vi "Dashboard Main.vi"(0 "Controller Type":string(combo)) -> ()   [LabVIEW 2020]
uses:
  <vilib>/Utility/miscctls.llb/LVRowAndColumnTypeDef.ctl
  <vilib>/event_ctls.llb/eventvkey.ctl
  <vilib>/Rock Robotics/Network Tables/NT Read Numeric Array.vi
  <vilib>/Rock Robotics/WPI/Dashboard/WPI_DashboardLogging Global.vi
panel:
  in  "Camera Settings Right":T1={"Frame Rate"=30, "Compression"=30, "Size"=1, "DB Camera Config"=FALSE} {"Frame Rate" scale=1.0..30.0; "Compression" scale=100.0..-1.0; "Size" items=["640x480", "320x240", "160x120"]}
  in  "Camera Name Right":string(combo)="No Camera Selection"
  out "Camera Perf":string
  in  "Camera Settings":T1={"Frame Rate"=30, "Compression"=30, "Size"=1, "DB Camera Config"=FALSE} {"Frame Rate" scale=1.0..30.0; "Compression" scale=100.0..-1.0; "Size" items=["640x480", "320x240", "160x120"]}
  in  "TCP":refnum<k5>
  in  "Rec Mode":enum32{"Stop", "Record", "Playback"}(radio)
  out "Robot IP":string
  out "Image Message":string="Timeout in Camera Communications"
  in  "Dashboard Tab":T2(tab)
  in  "Select Auto":string(combo)="Select Autonomous ..."
  out "NT Connection":bool
  out "MotorChart R":cluster{"Numeric":dbl, "Numeric":dbl}(graph)
  out "MotorChart L":cluster{"Numeric":dbl, "Numeric":dbl}(graph)
  out "MotorSliders R":cluster{"MotorSlide1":dbl, "MotorSlide2":dbl} {"MotorSlide2" scale=-1.0..1.0 scale format="%#_2e"; "MotorSlide1" scale=-1.0..1.0 scale format="%#_2e"}
  out "MotorSliders L":cluster{"MotorSlide1":dbl, "MotorSlide2":dbl} {"MotorSlide2" scale=-1.0..1.0 scale format="%#_2e"; "MotorSlide1" scale=-1.0..1.0 scale format="%#_2e"}
  out "Gyro":dbl(knob) scale=0.0..360.0
  out "JS1 Z":dbl(slide) scale=-1.0..1.0 scale format="%#_2e"
  out "JS1 Graph":cluster{"X":dbl, "Y":dbl}[](graph)
  out "JS1 Buttons":T3
  out "JS2 Z":dbl(slide) scale=-1.0..1.0 scale format="%#_2e"
  out "JS2 Graph":cluster{"X":dbl, "Y":dbl}[](graph)
  out "JS2 Buttons":T3
  out "Mode":T4(ring)=enum."Auto Disabled"
  out "Right Camera Perf":cluster{"Bandwidth (Mbps)":dbl, "FPS":dbl}
  out "Camera Image Right":T5(plugin-control)
  in  "DB/String 9":string
  in  "DB/String 8":string
  in  "DB/String 7":string
  in  "DB/String 6":string
  in  "DB/String 5":string
  in  "DB/String 4":string
  in  "DB/String 3":string
  in  "DB/String 2":string
  in  "DB/String 1":string
  in  "DB/String 0":string
  in  "DB/Slider 0":dbl(slide) scale=0.0..5.0
  in  "DB/Slider 1":dbl(slide) scale=0.0..5.0
  in  "DB/Slider 2":dbl(slide) scale=0.0..5.0
  in  "DB/Slider 3":dbl(slide) scale=0.0..5.0
  out "DB/LED 3":bool
  out "DB/LED 2":bool
  out "DB/LED 1":bool
  out "DB/LED 0":bool
  in  "DB/Button 3":bool
  in  "DB/Button 2":bool
  in  "DB/Button 1":bool
  in  "DB/Button 0":bool caption="New Name"
  out "Controller Verification":string
  in  "Test Slider":dbl(slide) scale=0.0..100.0 scale format="%#_3g"
  in  "On/Off":bool caption="Solenoid"
  in  "Test Name":u16(ring) items=["Select the test to run..."]
  in  "Test Tree":string(tree)
  in  "Motor":cluster{"Value":dbl, "Enable":bool} {"Value" scale=-1.0..1.0 scale format="%#_3g"}
  out "Progress":T6 {"Test Progress" scale=0.0..100.0}
  in  "Rev/Fwd":cluster{"Forward":bool, "Reverse":bool}
  in  "Test Ring":u16(ring) items=["Monochrome", "Color"]
  out "Cmd Status":string
  in  "Execute Command":bool
  in  "Command Params":string[][](table)
  in  "Command Selection":i32(listbox)
  in  "CheckList":i32(listbox)
  out "Tree":string(tree)
  out "Camera Image":T5(plugin-control)
  out "Background":bool
  in  "Camera Name":string(combo)="No Camera Selection"
  # "HW"
  # "HW"
  # "Joysticks"
  # "Drive Motors"
  # "Front"
  # "Right"
  # "Left"
  # "Back"
  # "This tab is a great place for autonomous settings and robot-specific values.\nPlace controls and indicators inside this tab and match name to\nDashboard Variables on robot. You can also delete this comment."
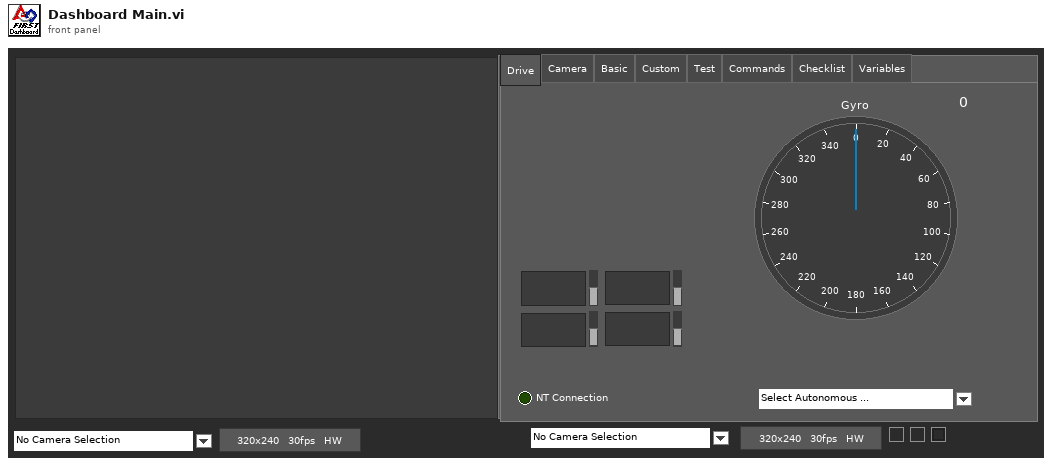
[diagram p1: front panel]
types:
  T1 = cluster{"Frame Rate":i32, "Compression":i32, "Size":u16, "DB Camera Config":bool}
  T2 = enum32{"Drive", "Camera", "Basic", "Custom", "Test", "Commands", "Checklist", "Variables"}
  T3 = cluster{bool, bool, bool, bool, bool, bool, bool, bool, bool, bool, bool, bool}
  T4 = enum8{"Tele-Op Disabled", "Tele-Op Enabled", "Auto Disabled", "Auto Enabled", "Test Disabled", "Test Enabled", "Disconnected", "No Code", "E-Stop"}
  T5 = typedef "IMAQ Image.ctl" = refnum<image>
  T6 = cluster{"Test Progress":u8, "Test Progress Text":string}
  T7 = cluster{"Save Path":path, "Interval (s)":dbl, "Keep":i32}
  T8 = typedef "Image Type" = u32
  T9 = cluster{"IDs":cluster{"RPC field ID":u16, "Unique ID":u16}, "String":string}
  T10 = cluster{"Error Strings":string, "Disable Counts":cluster{u16, u16}, "Rail Faults":cluster{u16, u16, u16}, "Robot IP":string, "DB Mode":u8, "Event Info":cluster{"Name":string, "Type":u8, "Number":u16, "Replay":u8}}
  T11 = cluster{"Storage":cluster{"Disk Free":u64, "RAM Block":u32, "RAM free":u32}, "CPU Utilization":cluster{"CPU % ISR":sgl, "CPU % Time Crit":sgl, "CPU % Timed Str":sgl, "CPU % High":sgl, "CPU % Above":sgl, "CPU % Normal":sgl, "CPU % Low":sgl}, "CAN":cluster{"% Bus Utilization":sgl, "Bus Off Cnt":u32, "TX_FIFO Full Cnt":u32, "Receive Error Cnt":u8, "Transmit Error Cnt":u8}, "HID":cluster{"HID Outputs":u32, "Rumble Low":u16, "Rumble High":u16}[]}
  T12 = cluster{"Status bits":cluster{"Test Mode":bool, "Autonomous":bool, "Enabled":bool, "Code Start":bool, "Brownout":bool, "Reserved 2":bool, "Reserved 3":bool, "E-Stop":bool}, "Code Trace":cluster{"Disabled":bool, "TeleOp":bool, "Auto":bool, "Test":bool}, "Controller Type":enum16{"unknown", "cRIO", "roboRio"}, "Code?":enum16{"unknown", "noCode", "code"}, "Battery V":dbl}
  T13 = cluster{"Control Bits":cluster{"TestMode":bool, "Autonomous":bool, "Enabled":bool, "FMS Present":bool, bool, bool, bool, "E-Stop":bool}, "Team Station ":u8, "Countdown":sgl, "Joystick Values":cluster{"Axes":dbl[], "Buttons":bool[], "POVs":i16[]}[]}
  T14 = cluster{"Axes":dbl[], "Buttons":bool[], "POVs":i16[]}[]
  T15 = cluster{"Axes":dbl[], "Buttons":bool[], "POVs":i16[]}
  T16 = cluster{"Buttons[0]":bool, "Buttons[1]":bool, "Buttons[2]":bool, "Buttons[3]":bool, "Buttons[4]":bool, "Buttons[5]":bool, "Buttons[6]":bool, "Buttons[7]":bool, "Buttons[8]":bool, "Buttons[9]":bool, "Buttons[10]":bool, "Buttons[11]":bool}
  T17 = cluster{"Camera Image":refnum<vi>, "Dashboard Tab":refnum<vi>, "Background":refnum<vi>, "Rec Mode":refnum<vi>, "Test Slider":refnum<vi>, "On/Off ":refnum<vi>, "Test Ring":refnum<vi>, "Rev/Fwd":refnum<vi>, "Test Name":refnum<vi>, "Motor":refnum<vi>, "Progress":refnum<vi>, "CheckList":refnum<vi>, "Tree":refnum<vi>, "Test Tree":refnum<vi>, "Command Params":refnum<vi>, "Command Selection":refnum<vi>, "Execute Command":refnum<vi>, "Cmd Status":refnum<vi>, "Camera Settings":refnum<vi>, "Camera Name":refnum<vi>, "Camera Perf":refnum<vi>, "Camera Settings Right":refnum<vi>, "Camera Name Right":refnum<vi>, "Camera Image Right":refnum<vi>}
  T18 = cluster{"Global Rectangle":i32[], "Contours":cluster{"Contour Type":u32, "ROI Type":u32, "Points":i32[]}[]}
  T19 = cluster{"Camera Name":string, string, "Saved DB Images Info":cluster{"Save Path":path, "Interval (s)":dbl, "Keep":i32}}
  T20 = cluster{"Camera Name Right":string, string, "Saved DB Images Info":cluster{"Save Path":path, "Interval (s)":dbl, "Keep":i32}}
  T21 = cluster{"Operation":enum16{"Update", "Clear"}, "Color Box":u32}[]
  T22 = typedef "eventvkey.ctl" = enum16{"ASCII", "Enter", "Return", "Shift", "Ctrl", "Alt", "Cmd", "Opt", "Caps", "NumLock", "Clear", "Break", "Up", "Down", "Left", "Right", "Insert", "Delete", "Home", "End", "PageUp", "PageDown", "Escape", "Help", "Pause", "ScrollLock", "F1", "F2", "F3", "F4", "F5", "F6", "F7", "F8", "F9", "F10", "F11", "F12", "F13", "F14", "F15", "F16", "F17", "F18", "F19", "F20", "F21", "F22", "F23", "F24", "Play", "VolumeUp", "VolumeDown", "Mute", "Two Byte Char"}
  T23 = cluster{"Image Size":bool, "Image Type":bool, "Pixel Value":bool, "ROI Information":bool, "Zoom Factor":bool}
  T24 = cluster{"Operation":enum16{"Update", "Clear"}, "Color Box":u32}
  T25 = typedef "LVRowAndColumnTypeDef.ctl" = cluster{"Row":i32, "Column":i32}
  T26 = cluster{"Shift":bool, "Ctrl":bool, "Alt":bool, "Cmd":bool, "Opt":bool}
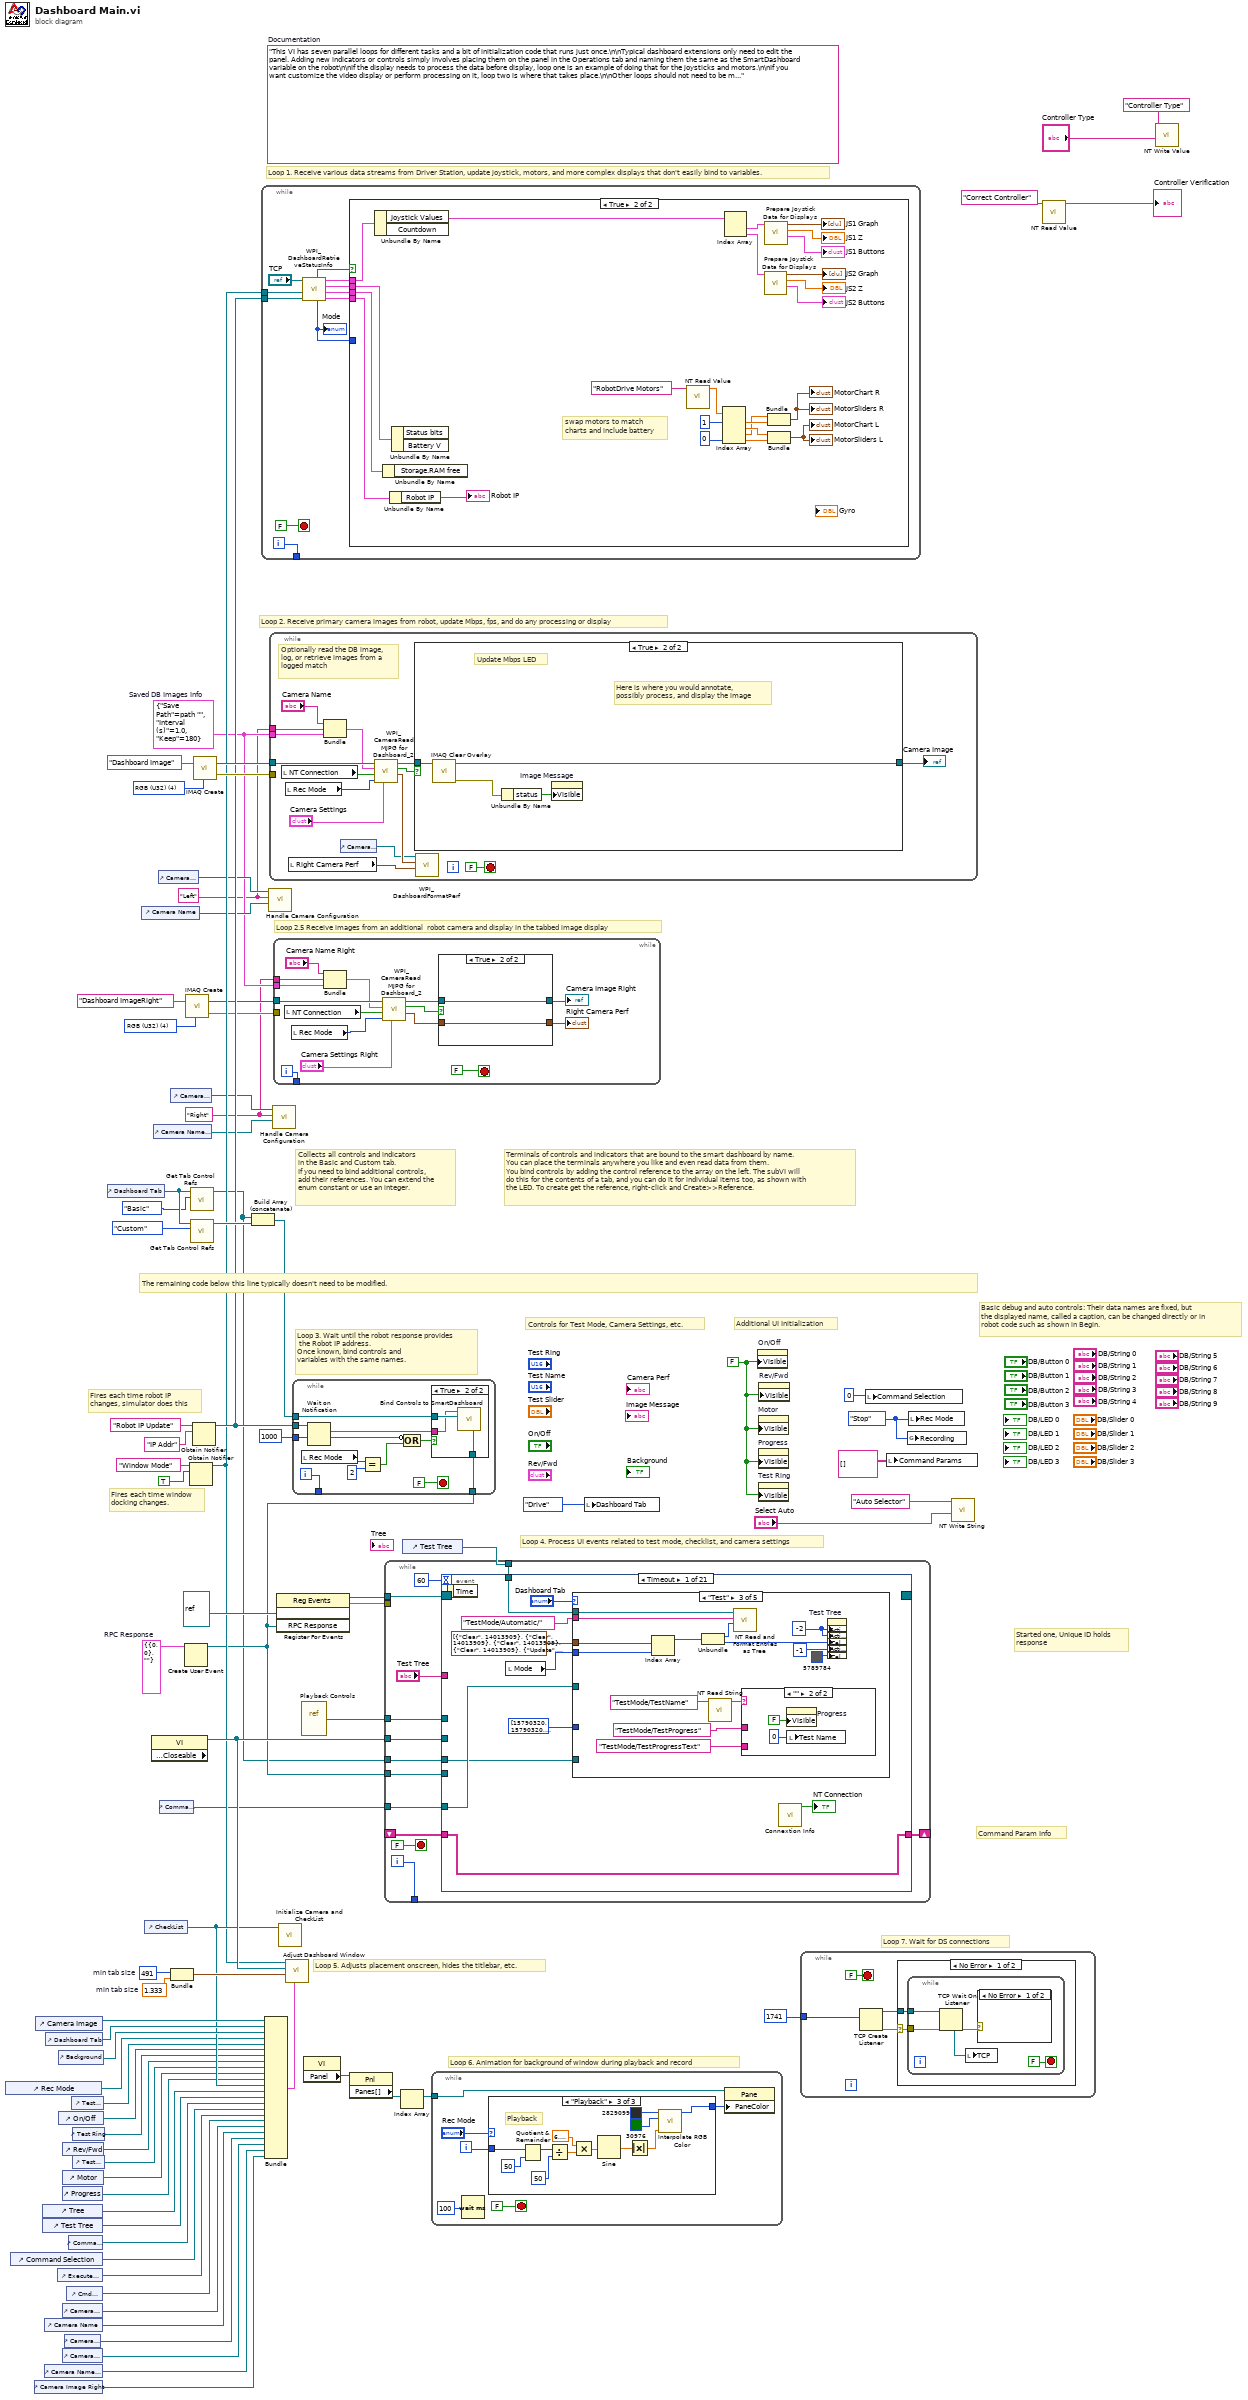
[diagram p0: block diagram]
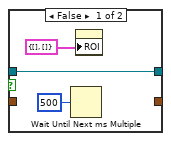
[diagram p2: hidden frame]
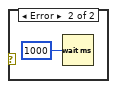
[diagram p3: hidden frame]
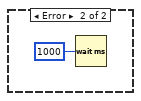
[diagram p4: hidden frame]
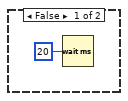
[diagram p5: hidden frame]
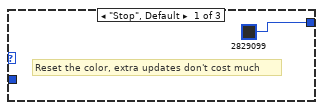
[diagram p6: hidden frame]
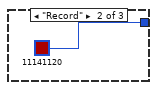
[diagram p7: hidden frame]
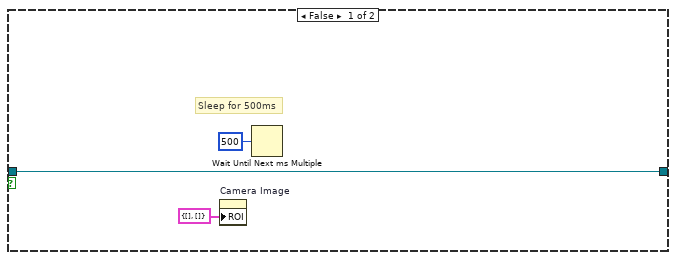
[diagram p9: hidden frame]
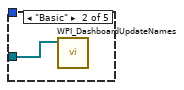
[diagram p11: hidden frame]
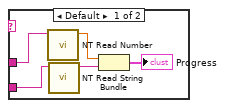
[diagram p12: hidden frame]
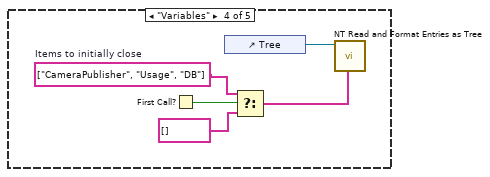
[diagram p13: hidden frame]
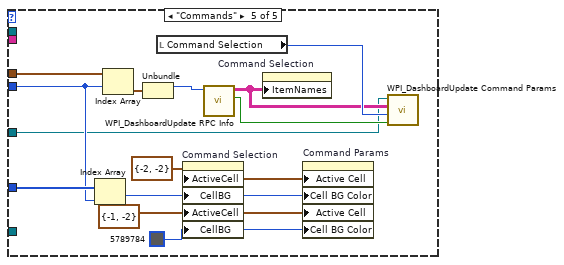
[diagram p14: hidden frame]
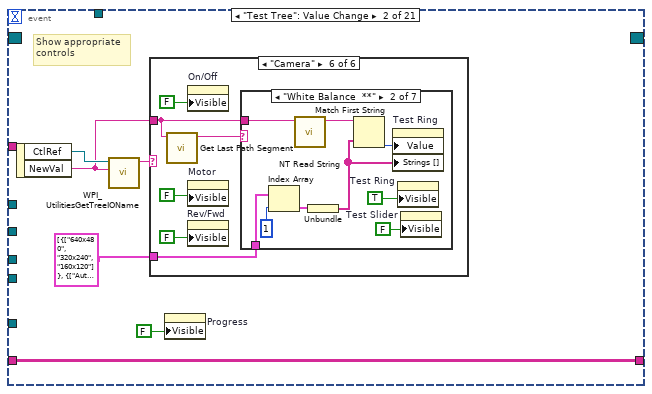
[diagram p15: hidden frame]
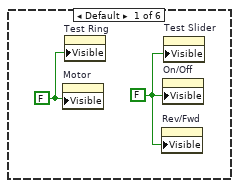
[diagram p16: hidden frame]
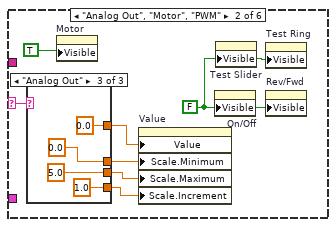
[diagram p17: hidden frame]
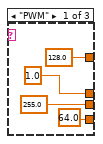
[diagram p18: hidden frame]
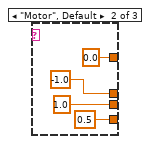
[diagram p19: hidden frame]
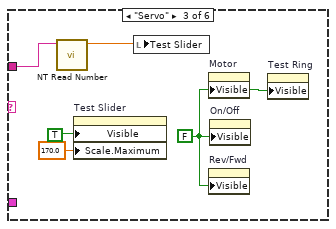
[diagram p20: hidden frame]
diagram:
  w7 = T7 {"Save Path"=path "", "Interval (s)"=1.0, "Keep"=180}  # Saved DB Images Info
  w6 = "Right"
  w5 = "Left"
  w17 = T8 4 items=["Grayscale (U8)", "Grayscale (I16)", "Grayscale (SGL)", "Complex (CSG)", "RGB (U32)", "HSL (U32)", "RGB (U64)"] ("Image Type")
  w33 = T9 {"IDs"={"RPC field ID"=0, "Unique ID"=0}, "String"=""}  # RPC Response
  w56 = 491  # min tab size
  w55 = 1.333  # min tab size
  w63 = enum32{"Stop", "Record", "Playback"}."Stop" ("Rec Mode")
  w40 = FALSE ("Visible")
  (unwired) "This VI has seven parallel loops for different tasks and a bit of initialization code that runs just once.\n\nTypical dashboard extensions only need to edit the panel. Adding new indicators or controls simply involves placing them on the panel in the Operations tab and naming them the same as the SmartDashboard variable on the robot\n\nIf the display needs to process the data before display, loop one is an example of doing that for the joysticks and motors.\n\nIf you want customize the video display or perform processing on it, loop two is where that takes place.\n\nOther loops should not need to be modified. They are pretty standard, and document the task they perform."  # Documentation
  w80 = T8 4 items=["Grayscale (U8)", "Grayscale (I16)", "Grayscale (SGL)", "Complex (CSG)", "RGB (U32)", "HSL (U32)", "RGB (U64)"] ("Image Type")
  # "Loop 2.5 Receive images from an additional  robot camera and display in the tabbed image display"
  # "Command Param Info"
  # "Started one, Unique ID holds\nresponse"
  # "Loop 7. Wait for DS connections"
  # "Basic debug and auto controls: Their data names are fixed, but\nthe displayed name, called a caption, can be changed directly or in\nrobot code such as shown in Begin."
  # "Controls for Test Mode, Camera Settings, etc."
  # "Additional UI Initialization"
  # "Loop 6. Animation for background of window during playback and record"
  # "Fires each time robot IP\nchanges, simulator does this"
  # "Fires each time window\ndocking changes."
  # "Collects all controls and indicators\nin the Basic and Custom tab.\nIf you need to bind additional controls,\nadd their references. You can extend the\nenum constant or use an integer."
  # "The remaining code below this line typically doesn't need to be modified."
  # "Loop 4. Process UI events related to test mode, checklist, and camera settings"
  # "Terminals of controls and indicators that are bound to the smart dashboard by name.\nYou can place the terminals anywhere you like and even read data from them.\nYou bind controls by adding the control reference to the array on the left. The subVI will\ndo this for the contents of a tab, and you can do it for individual items too, as shown with\nthe LED. To create get the reference, right-click and Create>>Reference."
  # "Loop 3. Wait until the robot response provides\n the Robot IP address.\nOnce known, bind controls and\nvariables with the same names."
  # "Loop 5. Adjusts placement onscreen, hides the titlebar, etc."
  # "Loop 1. Receive various data streams from Driver Station, update joystick, motors, and more complex displays that don't easily bind to variables."
  # "Loop 2. Receive primary camera images from robot, update Mbps, fps, and do any processing or display"
  n1 = control-ref of="Rec Mode"() -> (w46:refnum<vi>)
  n2 = control-ref of="Command Selection"() -> (w32:refnum<vi>)
  n3 = control-ref of="Camera Image Right"() -> (w10:refnum<vi>)
  n4 = control-ref of="Camera Image"() -> (w58:refnum<vi>)
  n5 = control-ref of="Tree"() -> (w50:refnum<vi>)
  n6 = control-ref of="Test Tree"() -> (w49:refnum<vi>)
  n7 = control-ref of="Camera Name"() -> (w23:refnum<vi>)
  n8 = control-ref of="Camera Name Right"() -> (w11:refnum<vi>)
  n9 = control-ref of="Dashboard Tab"() -> (w57:refnum<vi>)
  n10 = control-ref of="Execute Command"() -> (w34:refnum<vi>)
  n11 = control-ref of="Background"() -> (w53:refnum<vi>)
  n12 = control-ref of="On/Off"() -> (w44:refnum<vi>)
  n13 = control-ref of="Progress"() -> (w41:refnum<vi>)
  n14 = control-ref of="Camera Settings"() -> (w24:refnum<vi>)
  n15 = control-ref of="Camera Settings Right"() -> (w12:refnum<vi>)
  n16 = control-ref of="Rev/Fwd"() -> (w42:refnum<vi>)
  n17 = control-ref of="Motor"() -> (w47:refnum<vi>)
  n18 = control-ref of="Camera Perf"() -> (w22:refnum<vi>)
  n19 = control-ref of="Cmd Status"() -> (w28:refnum<vi>)
  n20 = control-ref of="Command Params"() -> (w35:refnum<vi>)
  n21 = control-ref of="Test Slider"() -> (w45:refnum<vi>)
  n22 = control-ref of="Test Ring"() -> (w43:refnum<vi>)
  n23 = control-ref of="Test Name"() -> (w48:refnum<vi>)
  n24 = control-ref of="Dashboard Tab"() -> (w61:refnum<vi>)
  n25 = control-ref of="Camera Name"() -> (w25:refnum<vi>)
  n26 = control-ref of="CheckList"() -> (w51:refnum<vi>)
  n27 = property class="VI" props=["Front Panel.Closeable"]() -> (reference out=w62:refnum<vi>)  [unwired: 2 in, 2 out]
  n28 = control-ref of="Camera Name Right"() -> (w13:refnum<vi>)
  n29 = control-ref of="Camera Settings"() -> (w26:refnum<vi>)
  n30 = control-ref of="Command Params"() -> (w27:refnum<vi>)
  n31 = control-ref of="Camera Settings Right"() -> (w14:refnum<vi>)
  n32 = Bundle("min tab size"=w56, "min tab size"=w55) -> (w54:cluster{"min tab size":i32, "min tab size":dbl})  [unwired: 1 in]
  n33 = Create User Event(user event datatype=w33) -> (user event=w29:refnum<user-event>)  [unwired: 1 in, 1 out]
  n34 = call "IMAQ Create"("Image Name"="Dashboard ImageRight", "Image Type"=w17) -> ("New Image"=w16:T5, "error out"=w15:errorcluster)  [unwired: 2 in, 1 out]
  n35 = Obtain Notifier(name (unnamed)="Window Mode", notification data type=TRUE) -> (notifier out=w38:refnum<notifier>)  [unwired: 2 in, 2 out]
  n36 = call <vilib>:"Get Tab Control Refs.vi"("Page Index"=T2."Basic" ("Dashboard Tab"), "TabControl in"=w61) -> ("ControlsOnPage"=w21:refnum<vi>[])  [unwired: 9 in]
  n37 = call <vilib>:"Get Tab Control Refs.vi"("Page Index"=T2."Custom" ("Dashboard Tab"), "TabControl in"=w61) -> ("ControlsOnPage"=w60:refnum<vi>[])  [unwired: 9 in]
  n38 = Obtain Notifier(name (unnamed)="Robot IP Update", notification data type="IP Addr" ("name (unnamed)")) -> (notifier out=w39:refnum<notifier>)  [unwired: 2 in, 2 out]
  n39 = call "IMAQ Create"("Image Name"="Dashboard Image", "Image Type"=w80) -> ("New Image"=w78:T5, "error out"=w77:errorcluster)  [unwired: 2 in, 1 out]
  n40 = Build Array (concatenate)(w21, w60) -> (w59:refnum<vi>[])
  n41 = while {
    tunnel: [w90] -> _
    tunnel: w39 -> [w84]
    tunnel: w38 -> [w81]
    i -> [w90]
    stop <- FALSE stop-if-true
    n42 = call <vilib>:"WPI_DashboardRetrieveStatusInfo.vi"("Binding Refnum"=w84, "Window Mode Notifier"=w81, "TCP Cnx"="TCP") -> ("Power and Errors"=w85:T10, "Robot Metrics"=w88:T11, "Status Info"=w89:T12, "Control Info"=w86:T13, "Robot Mode"=w83:T4, "Process?"=w87:bool)  [unwired: 3 in]
    "Mode" <- w83
    n43 = case shown="True" w87 {
      tunnel: w89 -> [_ w116]
      tunnel: w88 -> [_ w115]
      tunnel: w86 -> [_ w114]
      tunnel: w85 -> [_ w113]
      tunnel: w83 -> [_ _]
      frame False {
        n44 = Wait (ms)(milliseconds to wait=u32 20) -> ()  [unwired: 1 out]
      }
      frame True {
        # "swap motors to match\ncharts and include battery"
        n45 = Unbundle By Name(w114) -> ("Joystick Values"=w104:T14)  [unwired: 1 out]
        n46 = Unbundle By Name(w115) -> ()  [unwired: 1 out]
        n47 = Unbundle By Name(w113) -> ("Robot IP"=→"Robot IP":string)
        n48 = Unbundle By Name(w116) -> ()  [unwired: 2 out]
        n49 = call-poly <vilib>:"NT Read Value.vi"("Name"="RobotDrive Motors") -> ("Numeric Array"=w94:dbl[])  [unwired: 9 in, 1 out]
        n50 = Index Array(array=w94, index #1=1, index #4=0) -> (element #1=w108:dbl, element #2=w109:dbl, element #3=w107:dbl, element #4=w112:dbl)  [unwired: 2 in]
        n51 = Index Array(array=w104) -> (element #1=w103:T15, element #2=w99:T15)  [unwired: 2 in]
        n52 = call "Prepare Joystick Data for Displays.vi"("Joystick Values"=w99) -> ("Buttons"=→"JS2 Buttons":T16, "Z Axis"=→"JS2 Z":dbl, "Cartesian Data"=→"JS2 Graph":cluster{"X axis":dbl, "X axis":dbl}[])  [unwired: 8 in]
        n53 = call "Prepare Joystick Data for Displays.vi"("Joystick Values"=w103) -> ("Buttons"=→"JS1 Buttons":T16, "Z Axis"=→"JS1 Z":dbl, "Cartesian Data"=→"JS1 Graph":cluster{"X axis":dbl, "X axis":dbl}[])  [unwired: 8 in]
        n54 = Bundle("Numeric"=w107, "Numeric"=w108) -> (→"MotorChart R" →"MotorSliders R":cluster{"Numeric":dbl, "Numeric":dbl})  [unwired: 1 in]
        n55 = Bundle("Numeric"=w109, "Numeric"=w112) -> (→"MotorChart L" →"MotorSliders L":cluster{"Numeric":dbl, "Numeric":dbl})  [unwired: 1 in]
      }
    }
  }
  n56 = Bundle("Camera Image"=w58, "Dashboard Tab"=w57, "Background"=w53, "Rec Mode"=w46, "Test Slider"=w45, "On/Off"=w44, "Test Ring"=w43, "Rev/Fwd"=w42, "Test Name"=w48, "Motor"=w47, "Progress"=w41, "CheckList"=w51, "Tree"=w50, "Test Tree"=w49, "Command Params"=w35, "Command Selection"=w32, "Execute Command"=w34, "Cmd Status"=w28, "Camera Settings"=w24, "Camera Name"=w23, "Camera Perf"=w22, "Camera Settings Right"=w12, "Camera Name Right"=w11, "Camera Image Right"=w10) -> (w52:T17)  [unwired: 1 in]
  n57 = call "Handle Camera Configuration.vi"("CameraNameRef"=w25, "Display Name"=w5, "ClusterRef"=w26) -> ()  [unwired: 9 in]
  n58 = while {
    tunnel: w78 -> [w130]
    tunnel: w77 -> [_]
    tunnel: w7 -> [w123]
    tunnel: w5 -> [w120]
    stop <- FALSE stop-if-true
    # "Optionally read the DB image,\nlog, or retrieve images from a\nlogged match"
    n59 = local read "NT Connection"() -> (w124:bool)
    n60 = local read "Rec Mode"() -> (w127:enum32{"Stop", "Record", "Playback"})
    n61 = local read "Right Camera Perf"() -> (w118:cluster{"Bandwidth (Mbps)":dbl, "FPS":dbl})
    n62 = Bundle("Camera Name"="Camera Name", w120, "Saved DB Images Info"=w123) -> (w122:T19)  [unwired: 1 in]
    n63 = control-ref of="Camera Perf"() -> (w117:refnum<vi>)
    n64 = call <vilib>:"WPI_CameraRead MJPG for Dashboard_2.vi"("Camera Settings"="Camera Settings", "Rec Mode"=w127, "NT Connection"=w124, "Capture Info"=w122, "Image in"=w130) -> ("perf info"=w119:cluster{"Bandwidth (Mbps)":dbl, "fps":dbl}, "Active"=w128:bool, "Image\\ out"=w129:T5)  [unwired: 4 in]
    n65 = case shown="True" w128 {
      tunnel: w129 -> [w133 w136]
      tunnel: [w133 w135] -> w125
      frame False {
        # "Sleep for 500ms"
        n66 = property on="Camera Image" class="ImageControl"("ROI"=T18 {"Global Rectangle"=[], "Contours"=[]}) -> ()  [unwired: 2 in, 2 out]
        n67 = Wait Until Next ms Multiple(millisecond multiple=u32 500) -> ()  [unwired: 1 out]
      }
      frame True {
        # "Here is where you would annotate,\npossibly process, and display the image"
        # "Update Mbps LED"
        n68 = call "IMAQ Clear Overlay"("Image"=w136) -> ("error out"=w137:errorcluster, "Image Out"=w135:T5)  [unwired: 2 in, 7 out]
        n69 = Unbundle By Name(w137) -> ("status"=w138:bool)
        n70 = property on="Image Message" class="Str"("Visible"=w138) -> ()  [unwired: 2 in, 2 out]
      }
    }
    "Camera Image" <- w125
    n71 = call <vilib>:"WPI_DashboardFormatPerf.vi"("Right Camera Perf"=w118, "Performance"=w119, "String in"=w117) -> ()  [unwired: 9 in]
  }
  n72 = call "Handle Camera Configuration.vi"("CameraNameRef"=w13, "Display Name"=w6, "ClusterRef"=w14) -> ()  [unwired: 9 in]
  n73 = while {
    tunnel: w16 -> [w153]
    tunnel: w15 -> [_]
    tunnel: [w148] -> _
    tunnel: w7 -> [w144]
    tunnel: w6 -> [w141]
    i -> [w148]
    stop <- FALSE stop-if-true
    n74 = local read "NT Connection"() -> (w145:bool)
    n75 = local read "Rec Mode"() -> (w152:enum32{"Stop", "Record", "Playback"})
    n76 = Bundle("Camera Name Right"="Camera Name Right", w141, "Saved DB Images Info"=w144) -> (w143:T20)  [unwired: 1 in]
    n77 = call <vilib>:"WPI_CameraRead MJPG for Dashboard_2.vi"("Camera Settings"="Camera Settings Right", "Rec Mode"=w152, "NT Connection"=w145, "Capture Info"=w143, "Image in"=w153) -> ("perf info"=w139:cluster{"Bandwidth (Mbps)":dbl, "fps":dbl}, "Active"=w147:bool, "Image\\ out"=w150:T5)  [unwired: 4 in]
    n78 = case shown="True" w147 {
      tunnel: w150 -> [w155 w158]
      tunnel: [w155 w158] -> w146
      tunnel: [_ w157] -> w140
      tunnel: w139 -> [_ w157]
      frame False {
        n79 = Wait Until Next ms Multiple(millisecond multiple=u32 500) -> ()  [unwired: 1 out]
        n80 = property on="Camera Image Right" class="ImageControl"("ROI"=T18 {"Global Rectangle"=[], "Contours"=[]}) -> ()  [unwired: 2 in, 2 out]
      }
      frame True {
      }
    }
    "Camera Image Right" <- w146
    "Right Camera Perf" <- w140
  }
  n81 = register-events(refnum<vi> refnum, w29) -> (reference out=w67:refnum<event-registration>, error out=w66:errorcluster)  [unwired: 2 in]
  n82 = call "Initialize Camera and CheckList.vi"("ListBox in"=w51) -> ()  [unwired: 11 in]
  n83 = call "Adjust Dashboard Window.vi"("Sizing Refnums"=w52, "Size Constraints"=w54, "VI"=w62, "WIn Mode"=w38) -> ()  [unwired: 8 in]
  n84 = while {
    tunnel: w59 -> [w170]
    tunnel: w39 -> [w168]
    tunnel: [w166] -> _
    tunnel: u32 1000 ("milliseconds to wait") -> [w165]
    tunnel: w29 -> [w159]
    i -> [w166]
    stop <- FALSE stop-if-true
    n85 = local read "Rec Mode"() -> (w161:enum32{"Stop", "Record", "Playback"})
    n86 = Wait on Notification(notifier=w168, timeout in ms (-1)=w165) -> (notification=w167:string, timed out?=w163:bool)  [unwired: 2 in, 2 out]
    n87 = Equal?(x=w161, y=u16 2 ("Rec Mode")) -> (x = y?=w162:bool)
    n88 = Compound Arithmetic op=OR(invert w163, w162) -> (w164:bool)
    n89 = case shown="True" w164 {
      tunnel: w170 -> [_ w173]
      tunnel: w167 -> [_ w172]
      tunnel: w159 -> [_ w171]
      frame False {
      }
      frame True {
        n90 = call <vilib>:"Bind Controls to SmartDashboard.vi"("RPC ref"=w171, "Bound Control Refs"=w173, "Server IP Address"=w172) -> ()  [unwired: 9 in]
      }
    }
  }
  n91 = vi-ref "Playback Controls.vi"() -> (w68:refnum<vi>)
  n92 = property class="VI"() -> ("Panel"=w70:refnum<vi>)  [unwired: 2 in, 2 out]
  n93 = property class="Pnl"(reference=w70) -> ("Panes[]"=w71:refnum<vi>[])  [unwired: 1 in, 2 out]
  n94 = Index Array(array=w71) -> (element=w69:refnum<vi>)  [unwired: 1 in]
  n95 = control-ref of="Test Tree"() -> (w72:refnum<vi>)
  n96 = while {
    tunnel: [w183] -> _
    tunnel: w72 -> [w182]
    tunnel: w68 -> [w181]
    tunnel: w67 -> [w180]
    tunnel: w66 -> [_]
    tunnel: w62 -> [w179]
    tunnel: w29 -> [w178]
    tunnel: w27 -> [w177]
    shift-right: [w176] -> _
    shift-left: _ -> [w175]
    tunnel: w21 -> [w174]
    i -> [w183]
    stop <- FALSE stop-if-true
    n97 = event shown="[0] Timeout" {
      selector: w180 -> [_ _ _ _ _ _ _ _ _ _ _ _ _ _ _ _ _ _ _ _ _]
      dyn-events: [_ _ _ _ _ _ _ _ _ _ _ _ _ _ _ _ w443 _ _ _ _] -> _
      timeout: u32 60 ("milliseconds to wait") -> [_ _ _ _ _ _ _ _ _ _ _ _ _ _ _ _ _ _ _ _ _]
      tunnel: w182 -> [w195 _ _ _ _ _ _ _ _ _ _ _ _ _ _ _ _ _ _ _ _]
      tunnel: "Test Tree" -> [_ _ _ _ _ _ _ _ _ _ _ w410 w418 w420 w424 w432 _ _ _ _ _]
      tunnel: w181 -> [_ _ _ _ _ _ _ _ _ _ _ _ _ _ _ _ w445 _ w463 _ _]
      tunnel: w179 -> [_ _ _ _ _ _ _ _ _ _ _ _ _ _ _ _ w441 _ _ _ _]
      tunnel: w178 -> [_ _ _ _ _ _ _ _ _ _ _ _ _ _ _ _ w439 _ _ _ _]
      tunnel: w177 -> [w190 _ _ _ _ _ w361 _ _ _ _ _ _ _ _ _ _ _ _ _ _]
      tunnel: [w189 w238 w340 w345 w354 w358 w359 w368 w378 w385 w397 w409 w416 w419 w423 w431 w438 w458 w460 w464 w477] -> w176
      tunnel: w175 -> [w189 w238 w340 w345 w354 w358 w359 _ _ w385 w397 w409 w416 w419 w423 w431 w438 w458 w460 w464 w477]
      tunnel: w174 -> [w187 _ _ _ _ _ _ _ _ _ _ _ _ _ _ _ _ _ _ _ _]
      event Timeout {
        n98 = event-data() -> ()  [unwired: 1 in, 1 out]
        n99 = local read "Mode"() -> (w192:T4)
        n100 = case shown="\"Test\"" "Dashboard Tab" {
          tunnel: w195 -> [_ _ w211 _ _]
          tunnel: "TestMode/Automatic/" ("Name Pattern") -> [_ _ w210 _ _]
          tunnel: T21 [{"Operation"=enum."Clear", "Color Box"=14013909}, {"Operation"=enum."Clear", "Color Box"=14013909}, {"Operation"=enum."Clear", "Color Box"=14013909}, {"Operation"=enum."Clear", "Color Box"=14013909}, {"Operation"=enum."Update", "Color Box"=14013909}, {"Operation"=enum."Update", "Color Box"=16777215}, {"Operation"=enum."Clear", "Color Box"=14013909}, {"Operation"=enum."Clear", "Color Box"=14013909}, {"Operation"=enum."Clear", "Color Box"=14013909}] -> [_ _ w203 _ w231]
          tunnel: w192 -> [_ _ w202 _ w230]
          tunnel: u32[] [15790320, 15790320, 15790320, 15790320, 16777215, 16777215, 15790320, 15790320, 15790320] -> [_ _ _ _ w236]
          tunnel: w190 -> [_ _ _ _ w224]
          tunnel: w187 -> [_ w197 _ _ _]
          frame "Custom", Default {
          }
          frame "Basic" {
            n101 = call <vilib>:"WPI_DashboardUpdateNames.vi"("Controls on Tab"=w197) -> ()  [unwired: 11 in]
          }
          frame "Test" {
            w209 = -2 ("Active Item:Row Number")
            n102 = Index Array(array=w203, index=w202) -> (element=w204:T24)
            n103 = Unbundle(w204) -> ("Operation"=w205:enum16{"Update", "Clear"}, "Color Box"=w206:u32)
            n104 = call <vilib>:"NT Read String.vi"("Name"="TestMode/TestName") -> ("String"=w200:string)  [unwired: 9 in, 1 out]
            n105 = call <vilib>:"NT Read and Format Entries as Tree.vi"("Operation"=w205, "Name Pattern"=w210, "Tree Refnum"=w211) -> ()  [unwired: 7 in, 2 out]
            n106 = case shown="\"\"" w200 {
              tunnel: "TestMode/TestProgress" ("Name") -> [w213 _]
              tunnel: "TestMode/TestProgressText" ("Name") -> [w212 _]
              frame Default {
                n107 = call <vilib>:"NT Read Number.vi"("Name"=w213) -> ("Numeric"=w214:dbl)  [unwired: 9 in, 1 out]
                n108 = call <vilib>:"NT Read String.vi"("Name"=w212) -> ("String"=w215:string)  [unwired: 9 in, 1 out]
                n109 = Bundle("Numeric"=w214, "String"=w215) -> (→"Progress":cluster{"Numeric":dbl, "String":string})  [unwired: 1 in]
              }
              frame "" {
                n110 = property on="Progress" class="Clust (strict)"("Visible"=FALSE) -> ()  [unwired: 2 in, 2 out]
                n111 = local write "Test Name"(u16 0) -> ()
              }
            }
            n112 = property on="Test Tree" class="Tree (strict)"("Active Item Row Number"=w209, "ActiveColNum"=w209, "CellBG"=w206, "Active Item Row Number"=-1 ("Active Item:Row Number"), "CellBG"=u32 5789784 ("Color Box")) -> ()  [unwired: 2 in, 2 out]
          }
          frame "Variables" {
            w221 = string[] ["CameraPublisher", "Usage", "DB"]  # Items to initially close
            n113 = First Call?() -> (First Call?: T/F=w222:bool)
            n114 = control-ref of="Tree"() -> (w223:refnum<vi>)
            n115 = Select(t=w221, s=w222, f=string[] []) -> (s? t:f=w219:string[])
            n116 = call <vilib>:"NT Read and Format Entries as Tree.vi"("Tags to  Close"=w219, "Tree Refnum"=w223) -> ()  [unwired: 8 in, 2 out]
          }
          frame "Commands" {
            w232 = u32 5789784 ("Color Box")
            w233 = T25 {"Row"=-1, "Column"=-2} ("Active Cell:Active Cell")
            w235 = T25 {"Row"=-2, "Column"=-2} ("Active Cell:Active Cell")
            n117 = Index Array(array=w236, index=w230) -> (element=w234:u32)
            n118 = Index Array(array=w231, index=w230) -> (element=w229:T24)
            n119 = Unbundle(w229) -> ("Operation"=w228:enum16{"Update", "Clear"})  [unwired: 1 out]
            n120 = local read "Command Selection"() -> (w227:i32)
            n121 = property on="Command Selection" class="MCListbox (strict)"("ActiveCell"=w235, "CellBG"=w234, "ActiveCell"=w233, "CellBG"=w232) -> ()  [unwired: 2 in, 2 out]
            n122 = call <vilib>:"WPI_DashboardUpdate RPC Info.vi"("Operation"=w228) -> ("update"=w226:bool, "commands"=w225:string[][])  [unwired: 9 in]
            n123 = property on="Command Selection" class="MCListbox (strict)"("ItemNames"=w225) -> ()  [unwired: 2 in, 2 out]
            n124 = property on="Command Params" class="Tbl (strict)"("Active Cell"=w235, "Cell BG Color"=w234, "Active Cell"=w233, "Cell BG Color"=w232) -> ()  [unwired: 2 in, 2 out]
            n125 = call <vilib>:"WPI_DashboardUpdate Command Params.vi"("Update"=w226, "NewVal"=w227, "Commands"=w225, "Param Tbl"=w224) -> ()  [unwired: 7 in, 1 out]
          }
        }
        n126 = call <vilib>:"Connextion Info.vi"() -> ("Connected"=→"NT Connection":bool)  [unwired: 10 in, 1 out]
      }
      event "Test Tree": Value Change {
        # "Show appropriate\ncontrols"
        n127 = event-data() -> ("CtlRef"=w241:refnum<vi>, "NewVal"=w239:string)  [unwired: 1 in]
        n128 = call <vilib>:"WPI_UtilitiesGetTreeIOName.vi"("NewVal"=w239, "TreeControl in"=w241) -> ("I/O Name"=w242:string)  [unwired: 9 in]
        n129 = case shown="\"Camera\"" w242 {
          selector: w242 -> [_ w249 _ w271 w280 _]
          tunnel: w239 -> [_ _ w268 w270 _ w287]
          tunnel: cluster{string[]}[] [{["640x480", "320x240", "160x120"]}, {["Auto", "Fixed indoor", "Fixed outdoor 1", "Fixed outdoor 2", "Fixed fluorescent 1", "Fixed fluorescent 2", "Hold current"]}, {["Auto", "Flicker-free 50 Hz", "Flicker-free 60 Hz", "Hold current"]}, {["None", "Prioritize frame rate", "Prioritize image quality"]}, {["Monochrome", "Color"]}] -> [_ _ _ _ _ w286]
          frame Default {
            w244 = FALSE ("Visible")
            w243 = FALSE ("Visible")
            n130 = property on="Motor" class="Clust (strict)"("Visible"=w243) -> ()  [unwired: 2 in, 2 out]
            n131 = property on="Test Ring" class="Ring (strict)"("Visible"=w243) -> ()  [unwired: 2 in, 2 out]
            n132 = property on="Rev/Fwd" class="Clust (strict)"("Visible"=w244) -> ()  [unwired: 2 in, 2 out]
            n133 = property on="On/Off" class="Bool (strict)"("Visible"=w244) -> ()  [unwired: 2 in, 2 out]
            n134 = property on="Test Slider" class="Slide (strict)"("Visible"=w244) -> ()  [unwired: 2 in, 2 out]
          }
          frame "Analog Out", "Motor", "PWM" {
            w250 = FALSE ("Visible")
            n135 = case shown="\"Analog Out\"" w249 {
              tunnel: [1.0 ("Value") -1.0 ("Value") 0.0 ("Value")] -> w248
              tunnel: [255.0 ("Value") 1.0 ("Value") 5.0 ("Value")] -> w247
              tunnel: [128.0 ("Value") 0.0 ("Value") 0.0 ("Value")] -> w246
              tunnel: [64.0 ("Value") 0.5 ("Value") 1.0 ("Value")] -> w245
              frame "PWM" {
              }
              frame "Motor", Default {
              }
              frame "Analog Out" {
              }
            }
            n136 = property on="Motor" class="Clust (strict)"("Visible"=TRUE) -> ()  [unwired: 2 in, 2 out]
            n137 = property on="Value" class="Slide (strict)"("Value"=w246, "Scale.Minimum"=w248, "Scale.Maximum"=w247, "Scale.Increment"=w245) -> ()  [unwired: 2 in, 2 out]
            n138 = property on="On/Off" class="Bool (strict)"("Visible"=w250) -> ()  [unwired: 2 in, 2 out]
            n139 = property on="Test Slider" class="Slide (strict)"("Visible"=w250) -> ()  [unwired: 2 in, 2 out]
            n140 = property on="Test Ring" class="Ring (strict)"("Visible"=w250) -> ()  [unwired: 2 in, 2 out]
            n141 = property on="Rev/Fwd" class="Clust (strict)"("Visible"=w250) -> ()  [unwired: 2 in, 2 out]
          }
          frame "Servo" {
            w266 = FALSE ("Visible")
            n142 = call <vilib>:"NT Read Number.vi"("Name"=w268) -> ("Numeric"=w267:dbl)  [unwired: 9 in, 1 out]
            n143 = property on="Test Slider" class="Slide (strict)"("Visible"=TRUE, "Scale.Maximum"=170.0 ("Scale.Range:Maximum")) -> ()  [unwired: 2 in, 2 out]
            n144 = local write "Test Slider"(w267) -> ()
            n145 = property on="Motor" class="Clust (strict)"("Visible"=w266) -> ()  [unwired: 2 in, 2 out]
            n146 = property on="Rev/Fwd" class="Clust (strict)"("Visible"=w266) -> ()  [unwired: 2 in, 2 out]
            n147 = property on="On/Off" class="Bool (strict)"("Visible"=w266) -> ()  [unwired: 2 in, 2 out]
            n148 = property on="Test Ring" class="Ring (strict)"("Visible"=w266) -> ()  [unwired: 2 in, 2 out]
          }
          frame "Relay", "Solenoid" {
            w269 = FALSE ("Visible")
            n149 = property on="Motor" class="Clust (strict)"("Visible"=w269) -> ()  [unwired: 2 in, 2 out]
            n150 = property on="Test Slider" class="Slide (strict)"("Visible"=w269) -> ()  [unwired: 2 in, 2 out]
            n151 = Search and Replace String(input string=w270, search string="/Value  **", replace string="/Direction") -> (result string=w276:string)  [unwired: 5 in, 3 out]
            n152 = property on="Test Ring" class="Ring (strict)"("Visible"=w269) -> ()  [unwired: 2 in, 2 out]
            n153 = call <vilib>:"NT Read String.vi"("Name"=w276) -> ("String"=w274:string)  [unwired: 9 in, 1 out]
            n154 = Equal?(x="Both directions", y=w274) -> (x = y?=w272:bool)
            n155 = Not(x=w272) -> (.not. x?=w273:bool)
            n156 = property on="Rev/Fwd" class="Clust (strict)"("Visible"=w272) -> ()  [unwired: 2 in, 2 out]
            n157 = property on="On/Off" class="Bool (strict)"("Visible"=w273, "Caption.Text"=w271) -> ()  [unwired: 2 in, 2 out]
          }
          frame "Compressor", "Digital Out" {
            w279 = FALSE ("Visible")
            # "Get direction and finish"
            n158 = property on="Motor" class="Clust (strict)"("Visible"=w279) -> ()  [unwired: 2 in, 2 out]
            n159 = property on="Test Slider" class="Slide (strict)"("Visible"=w279) -> ()  [unwired: 2 in, 2 out]
            n160 = property on="Test Ring" class="Ring (strict)"("Visible"=w279) -> ()  [unwired: 2 in, 2 out]
            n161 = property on="On/Off" class="Bool (strict)"("Visible"=TRUE, "Caption.Text"=w280) -> ()  [unwired: 2 in, 2 out]
            n162 = property on="Rev/Fwd" class="Clust (strict)"("Visible"=FALSE) -> ()  [unwired: 2 in, 2 out]
          }
          frame "Camera" {
            n163 = call <vilib>:"Get Last Path Segment.vi"("String in"=w287) -> ("String out"=w288:string)  [unwired: 10 in]
            n164 = property on="On/Off" class="Bool (strict)"("Visible"=FALSE) -> ()  [unwired: 2 in, 2 out]
            n165 = property on="Motor" class="Clust (strict)"("Visible"=FALSE) -> ()  [unwired: 2 in, 2 out]
            n166 = property on="Rev/Fwd" class="Clust (strict)"("Visible"=FALSE) -> ()  [unwired: 2 in, 2 out]
            n167 = case shown="\"White Balance  **\"" w288 {
              tunnel: w287 -> [w294 w303 w312 w321 w330 _ w336]
              tunnel: w286 -> [w292 w300 w309 w318 w327 _ _]
              frame "Size  **" {
                n168 = Index Array(array=w292) -> (element=w291:cluster{string[]})  [unwired: 1 in]
                n169 = call <vilib>:"NT Read String.vi"("Name"=w294) -> ("String"=w293:string)  [unwired: 9 in, 1 out]
                n170 = Unbundle(w291) -> (w289:string[])
                n171 = Match First String(2:w289, 3:w293) -> (0:w290:i32)  [unwired: 1 out]
                n172 = property on="Test Ring" class="Ring (strict)"("Value"=w290, "Strings []"=w289) -> ()  [unwired: 2 in, 2 out]
                n173 = property on="Test Ring" class="Ring (strict)"("Visible"=TRUE) -> ()  [unwired: 2 in, 2 out]
                n174 = property on="Test Slider" class="Slide (strict)"("Visible"=FALSE) -> ()  [unwired: 2 in, 2 out]
              }
              frame "White Balance  **" {
                n175 = Index Array(array=w300, index=1) -> (element=w301:cluster{string[]})
                n176 = call <vilib>:"NT Read String.vi"("Name"=w303) -> ("String"=w302:string)  [unwired: 9 in, 1 out]
                n177 = Unbundle(w301) -> (w298:string[])
                n178 = Match First String(2:w298, 3:w302) -> (0:w297:i32)  [unwired: 1 out]
                n179 = property on="Test Ring" class="Ring (strict)"("Value"=w297, "Strings []"=w298) -> ()  [unwired: 2 in, 2 out]
                n180 = property on="Test Ring" class="Ring (strict)"("Visible"=TRUE) -> ()  [unwired: 2 in, 2 out]
                n181 = property on="Test Slider" class="Slide (strict)"("Visible"=FALSE) -> ()  [unwired: 2 in, 2 out]
              }
              frame "Exposure  **" {
                n182 = Index Array(array=w309, index=2) -> (element=w310:cluster{string[]})
                n183 = call <vilib>:"NT Read String.vi"("Name"=w312) -> ("String"=w311:string)  [unwired: 9 in, 1 out]
                n184 = Unbundle(w310) -> (w306:string[])
                n185 = Match First String(2:w306, 3:w311) -> (0:w307:i32)  [unwired: 1 out]
                n186 = property on="Test Ring" class="Ring (strict)"("Value"=w307, "Strings []"=w306) -> ()  [unwired: 2 in, 2 out]
                n187 = property on="Test Ring" class="Ring (strict)"("Visible"=TRUE) -> ()  [unwired: 2 in, 2 out]
                n188 = property on="Test Slider" class="Slide (strict)"("Visible"=FALSE) -> ()  [unwired: 2 in, 2 out]
              }
              frame "Exposure Priority  **" {
                n189 = Index Array(array=w318, index=3) -> (element=w319:cluster{string[]})
                n190 = call <vilib>:"NT Read String.vi"("Name"=w321) -> ("String"=w320:string)  [unwired: 9 in, 1 out]
                n191 = Unbundle(w319) -> (w315:string[])
                n192 = Match First String(2:w315, 3:w320) -> (0:w316:i32)  [unwired: 1 out]
                n193 = property on="Test Ring" class="Ring (strict)"("Value"=w316, "Strings []"=w315) -> ()  [unwired: 2 in, 2 out]
                n194 = property on="Test Ring" class="Ring (strict)"("Visible"=TRUE) -> ()  [unwired: 2 in, 2 out]
                n195 = property on="Test Slider" class="Slide (strict)"("Visible"=FALSE) -> ()  [unwired: 2 in, 2 out]
              }
              frame "Color Enable  **" {
                n196 = Index Array(array=w327, index=4) -> (element=w328:cluster{string[]})
                n197 = call <vilib>:"NT Read String.vi"("Name"=w330) -> ("String"=w329:string)  [unwired: 9 in, 1 out]
                n198 = Unbundle(w328) -> (w324:string[])
                n199 = Match First String(2:w324, 3:w329) -> (0:w325:i32)  [unwired: 1 out]
                n200 = property on="Test Ring" class="Ring (strict)"("Value"=w325, "Strings []"=w324) -> ()  [unwired: 2 in, 2 out]
                n201 = property on="Test Ring" class="Ring (strict)"("Visible"=TRUE) -> ()  [unwired: 2 in, 2 out]
                n202 = property on="Test Slider" class="Slide (strict)"("Visible"=FALSE) -> ()  [unwired: 2 in, 2 out]
              }
              frame Default {
                n203 = property on="Test Ring" class="Ring (strict)"("Visible"=FALSE) -> ()  [unwired: 2 in, 2 out]
                n204 = property on="Test Slider" class="Slide (strict)"("Visible"=FALSE) -> ()  [unwired: 2 in, 2 out]
              }
              frame "Brightness  **", "Color Level  **", "Compression  **", "FPS  **", "Sharpness  **" {
                n205 = call <vilib>:"NT Read Number.vi"("Name"=w336) -> ("Numeric"=w335:dbl)  [unwired: 9 in, 1 out]
                n206 = local write "Test Slider"(w335) -> ()
                n207 = property on="Test Slider" class="Slide (strict)"("Visible"=TRUE, "Scale.Maximum"=100.0 ("Scale.Range:Maximum")) -> ()  [unwired: 2 in, 2 out]
                n208 = property on="Test Ring" class="Ring (strict)"("Visible"=FALSE) -> ()  [unwired: 2 in, 2 out]
              }
            }
          }
        }
        n209 = property on="Progress" class="Clust (strict)"("Visible"=FALSE) -> ()  [unwired: 2 in, 2 out]
      }
      event "Test Name": Mouse Enter {
        # "Populate the ring with the list of tests"
        n210 = event-data() -> ()  [unwired: 1 in, 1 out]
        n211 = call <vilib>:"NT Read String Array.vi"("Name"="TestMode/TestList") -> ("String Array"=w344:string[])  [unwired: 9 in, 1 out]
        n212 = Build Array (concatenate)("Select the test to run...", w344) -> (w343:string[])
        n213 = property on="Test Name" class="Ring (strict)"("Strings []"=w343) -> ()  [unwired: 2 in, 2 out]
      }
      event "Test Name": Value Change {
        w346 = FALSE ("Visible")
        # "Tell the robot the test name to run"
        n214 = event-data() -> ("NewVal"=w350:u16)  [unwired: 1 in]
        n215 = property on="Test Name" class="Ring (strict)"() -> ("Strings []"=w351:string[])  [unwired: 2 in, 2 out]
        n216 = local write "Progress"(T6 {"Test Progress"=0, "Test Progress Text"=""} ("Progress")) -> ()
        n217 = Index Array(array=w351, index=w350) -> (element=w349:string)
        n218 = call <vilib>:"NT Write String.vi"("String"=w349, "Name"="TestMode/TestName") -> ()  [unwired: 9 in, 1 out]
        n219 = property on="Progress" class="Clust (strict)"("Visible"=TRUE) -> ()  [unwired: 2 in, 2 out]
        n220 = property on="Motor" class="Clust (strict)"("Visible"=w346) -> ()  [unwired: 2 in, 2 out]
        n221 = property on="Test Slider" class="Slide (strict)"("Visible"=w346) -> ()  [unwired: 2 in, 2 out]
        n222 = property on="On/Off" class="Bool (strict)"("Visible"=w346) -> ()  [unwired: 2 in, 2 out]
        n223 = property on="Rev/Fwd" class="Clust (strict)"("Visible"=w346) -> ()  [unwired: 2 in, 2 out]
        n224 = property on="Test Ring" class="Ring (strict)"("Visible"=w346) -> ()  [unwired: 2 in, 2 out]
      }
      event "Select Auto": Mouse Enter {
        # "Populate the combo box with the list of autonomous options"
        n225 = event-data() -> ()  [unwired: 1 in, 1 out]
        n226 = call <vilib>:"NT Read String Array.vi"("Name"="Auto List") -> ("String Array"=w353:string[])  [unwired: 9 in, 1 out]
        n227 = property on="Select Auto" class="CmbBox"("Strings[]"=w353) -> ()  [unwired: 2 in, 2 out]
      }
      event "Select Auto": Value Change {
        # "User modified the Auto Selection. Write to NT variable so robot knows."
        n228 = event-data() -> ("NewVal"=w356:string)  [unwired: 1 in]
        n229 = call <vilib>:"NT Write String.vi"("String"=w356, "Name"="Auto Selector") -> ()  [unwired: 9 in, 1 out]
      }
      event "Command Selection": Value Change {
        # "Get the params and show in table"
        n230 = event-data() -> ("NewVal"=w362:i32)  [unwired: 1 in]
        n231 = property on="Command Selection" class="MCListbox (strict)"() -> ("ItemNames"=w360:string[][])  [unwired: 2 in, 2 out]
        n232 = call <vilib>:"WPI_DashboardUpdate Command Params.vi"("NewVal"=w362, "Commands"=w360, "Param Tbl"=w361) -> ()  [unwired: 8 in, 1 out]
      }
      event "Execute Command": Value Change {
        # "Started one, Unique ID holds\nresponse"
        n233 = event-data() -> ()  [unwired: 1 in, 1 out]
        n234 = property on="Command Selection" class="MCListbox (strict)"() -> ("ItemNames"=w373:string[][])  [unwired: 2 in, 2 out]
        n235 = Index Array(array=w373, index (row)="Command Selection", index (col)=0) -> (element=w371:string)
        n236 = call <vilib>:"Invoke Commands.vi"("Command Params"="Command Params", "Function Name"=w371) -> ("Params"=w367:u8, "Started"=w366:bool)  [unwired: 7 in, 1 out]
        n237 = Array Subset(array="Command Params", length (row)=w367) -> (w368:string[][])  [unwired: 3 in]
        n238 = Select(t="Executing" ("Cmd Status"), s=w366, f="" ("Cmd Status")) -> (s? t:f=→"Cmd Status":string)
      }
      event "Command Selection": Double Click {
        n239 = event-data() -> ("Row"=w381:i32)  [unwired: 1 in]
        n240 = property on="Command Selection" class="MCListbox (strict)"() -> ("ItemNames"=w384:string[][])  [unwired: 2 in, 2 out]
        n241 = local read "Command Params"() -> (w380:string[][])
        n242 = Index Array(array=w384, index (row)=w381, index (col)=0) -> (element=w382:string)
        n243 = call <vilib>:"Invoke Commands.vi"("Command Params"=w380, "Function Name"=w382) -> ("Params"=w379:u8, "Started"=w374:bool)  [unwired: 7 in, 1 out]
        n244 = Array Subset(array=w380, length (row)=w379) -> (w378:string[][])  [unwired: 3 in]
        n245 = Select(t="Executing" ("Cmd Status"), s=w374, f="" ("Cmd Status")) -> (s? t:f=w375:string)
        n246 = local write "Cmd Status"(w375) -> ()
      }
      event "CheckList": Double Click {
        # "Shift clears all"
        # "Update symbols on the listbox"
        n247 = event-data() -> ("PlatMods.Shift"=w386:bool, "Row"=w388:i32)  [unwired: 1 in]
        n248 = case shown="True" w386 {
          tunnel: w388 -> [w392 _]
          tunnel: 1 -> [w391 _]
          frame False {
            n249 = property on="CheckList" class="LstBox (strict)"() -> ("Item Symbols"=w390:i32[])  [unwired: 2 in, 2 out]
            n250 = Replace Array Subset(array=w390, new element=w391, index=w392) -> (w389:i32[])
            n251 = property on="CheckList" class="LstBox (strict)"("Item Symbols"=w389) -> ()  [unwired: 2 in, 2 out]
          }
          frame True {
            w393 = 0 ("Top Row")
            n252 = property on="CheckList" class="LstBox (strict)"() -> ("Number of Rows"=w395:u32)  [unwired: 2 in, 2 out]
            n253 = Initialize Array(0, w395) -> (w394:i32[])
            n254 = property on="CheckList" class="LstBox (strict)"("Top Row"=w393, "Value"=w393, "Item Symbols"=w394) -> ()  [unwired: 2 in, 2 out]
          }
        }
      }
      event "CheckList": Key Down {
        # "Update symbols on the listbox\nLeft and right keys check and uncheck"
        n255 = event-data() -> ("VKey"=w399:T22)  [unwired: 1 in]
        n256 = case shown="\"Left\", \"Right\"" w399 {
          selector: w399 -> [w404 _]
          tunnel: eventvkey."Left" ("VKey") -> [w402 _]
          frame "Left", "Right" {
            n257 = Equal?(x=w402, y=w404) -> (x = y?=w403:bool)
            n258 = Select(t=0, s=w403, f=1) -> (s? t:f=w405:i32)
            n259 = property on="CheckList" class="LstBox (strict)"() -> ("Item Symbols"=w408:i32[])  [unwired: 2 in, 2 out]
            n260 = Replace Array Subset(array=w408, new element=w405, index="CheckList") -> (w407:i32[])
            n261 = property on="CheckList" class="LstBox (strict)"("Item Symbols"=w407) -> ()  [unwired: 2 in, 2 out]
          }
          frame Default {
          }
        }
      }
      event "Motor.Enable": Value Change {
        # "When the test mode otor enable helper is set, update that\ntree row item's value"
        n262 = event-data() -> ("NewVal"=w414:bool)  [unwired: 1 in]
        n263 = Unbundle("Motor") -> ("Value"=w413:dbl)  [unwired: 1 out]
        n264 = Select(t=w413, s=w414, f=0.0) -> (s? t:f=w411:dbl)
        n265 = call <vilib>:"NT Write Number.vi"("Numeric"=w411, "Name"=w410) -> ()  [unwired: 9 in, 1 out]
      }
      event "Test Slider": Value Change {
        # "When the test mode slider helper is set, update that\ntree row item's value"
        n266 = event-data() -> ("NewVal"=w417:dbl)  [unwired: 1 in]
        n267 = call <vilib>:"NT Write Number.vi"("Numeric"=w417, "Name"=w418) -> ()  [unwired: 9 in, 1 out]
      }
      event "On/Off": Value Change {
        # "When the test mode on/off helper value is set, update that\ntree row item's value"
        n268 = event-data() -> ("NewVal"=w422:bool)  [unwired: 1 in]
        n269 = Boolean To (0,1)(Boolean=w422) -> (0, 1=w421:i16)
        n270 = call <vilib>:"NT Write Number.vi"("Numeric"=w421, "Name"=w420) -> ()  [unwired: 9 in, 1 out]
      }
      event "Rev/Fwd": Value Change {
        # "When the test mode helper value for relays is set, update that\ntree row item's value"
        n271 = event-data() -> ("NewVal.Forward"=w430:bool, "NewVal.Reverse"=w429:bool)  [unwired: 1 in]
        n272 = Boolean To (0,1)(Boolean=w430) -> (0, 1=w426:i16)
        n273 = Boolean To (0,1)(Boolean=w429) -> (0, 1=w428:i16)
        n274 = Negate(x=w428) -> (-x=w427:i16)
        n275 = Add(x=w426, y=w427) -> (x+y=w425:i16)
        n276 = call <vilib>:"NT Write Number.vi"("Numeric"=w425, "Name"=w424) -> ()  [unwired: 9 in, 1 out]
      }
      event "Test Ring": Value Change {
        # "When a test mode helper value is selected from the ring,\nset the tree item's variable to the string value"
        n277 = event-data() -> ("NewVal"=w434:u16)  [unwired: 1 in]
        n278 = property on="Test Ring" class="Ring (strict)"() -> ("Strings []"=w435:string[])  [unwired: 2 in, 2 out]
        n279 = Index Array(array=w435, index=w434) -> (element=w433:string)
        n280 = call <vilib>:"NT Write String.vi"("String"=w433, "Name"=w432) -> ()  [unwired: 9 in, 1 out]
      }
      event "Rec Mode": Value Change {
        # "Update globals for recording mode and path to read log from.\nClear when logging and let NetworkTables set path for vision to\nuse."
        n281 = event-data() -> ("NewVal"=w446:enum32{"Stop", "Record", "Playback"})  [unwired: 1 in]
        n282 = global write "WPI_DashboardLogging Global.vi" "Logging Filename"(path "") -> ()
        n283 = global write "WPI_DashboardLogging Global.vi" "Recording"(w446) -> ()
        n284 = case shown="\"Playback\"" w446 {
          tunnel: w445 -> [_ w448 w457]
          tunnel: [_ _ w456] -> w443
          tunnel: [_ _ w455] -> _
          tunnel: w441 -> [_ _ w453]
          tunnel: cluster{i32, i32} {-250, 170} -> [_ _ w452]
          tunnel: [_ _ T23 {"Image Size"=TRUE, "Image Type"=TRUE, "Pixel Value"=TRUE, "ROI Information"=TRUE, "Zoom Factor"=FALSE} ("Image Information Shown:All Elements")] -> w436
          tunnel: [_ _ TRUE ("Zoom Factor")] -> w437
          tunnel: w439 -> [_ _ w449]
          frame Default {
          }
          frame "Stop", "Record" {
            # "Place Window too"
            n285 = invoke class="VI" method="FP.Close"(reference=w448) -> (reference out=w447:refnum<vi>)  [unwired: 2 in, 2 out]
            n286 = invoke class="VI" method="Abort VI"(reference=w447) -> ()  [unwired: 2 in, 3 out]
          }
          frame "Playback" {
            n287 = call "Open Playback Panel.vi"("Offset"=w452, "DB VI Ref"=w453, "Playback in"=w457) -> ("Playback out"=w454:refnum<vi>)  [unwired: 8 in]
            n288 = register-events(w454, w449) -> (reference out=w456:refnum<event-registration>, error out=w455:errorcluster)  [unwired: 2 in]
          }
        }
        n289 = property on="Camera Image Right" class="ImageControl"("Image Information Shown"=w436, "Image Information Visible"=w437) -> ()  [unwired: 2 in, 2 out]
        n290 = property on="Camera Image" class="ImageControl"("Image Information Shown"=w436, "Image Information Visible"=w437) -> ()  [unwired: 2 in, 2 out]
        n291 = call <vilib>:"WPI_DashboardNT Log FieldName Cache.vi"("Operation"=enum16{"Lookup/Add", "Index", "Clear"}."Clear") -> ()  [unwired: 8 in, 3 out]
      }
      event Panel Close {
        w459 = enum32{"Stop", "Record", "Playback"}."Stop" ("Rec Mode")
        # "Playback window has been closed, abort"
        n292 = event-data() -> ()  [unwired: 1 in, 4 out]
        n293 = local write "Rec Mode"(w459) -> ()
        n294 = global write "WPI_DashboardLogging Global.vi" "Recording"(w459) -> ()
      }
      event Panel Close {
        # "Abort playback window and ourself"
        n295 = event-data() -> ()  [unwired: 1 in, 4 out]
        n296 = invoke class="VI" method="FP.Close"(reference=w463) -> (reference out=w462:refnum<vi>)  [unwired: 2 in, 2 out]
        n297 = invoke class="VI" method="Abort VI"(reference=w462) -> (error out=w461:errorcluster)  [unwired: 2 in, 2 out]
        n298 = invoke class="VI" method="Abort VI"(error in=w461) -> ()  [unwired: 2 in, 3 out]
      }
      event User Event {
        n299 = event-data() -> ("IDs"=w470:cluster{"RPC field ID":u16, "Unique ID":u16}, "String"=w469:string)  [unwired: 1 in]
        n300 = Bundle("IDs"=w470, "String"=w469) -> (w468:T9)  [unwired: 1 in]
        n301 = call <vilib>:"Retrieve RPC Response.vi"("RPC Response"=w468) -> ("Output"=w466:string[][])  [unwired: 10 in]
        n302 = Build Array (concatenate)(w464, w466) -> (w465:string[][])
        n303 = local write "Command Params"(w465) -> ()
        n304 = local write "Cmd Status"("" ("Cmd Status")) -> ()
      }
      event "Tree": Double Click {
        n305 = event-data() -> ("PlatMods"=w476:T26, "Tag"=w473:string)  [unwired: 1 in]
        n306 = Unbundle(w476) -> ("Shift"=w475:bool)  [unwired: 4 out]
        n307 = String Subset(string=w473, length (rest)=1 ("length (rest)")) -> (substring=w472:string)  [unwired: 1 in]
        n308 = Not(x=w475) -> (.not. x?=w474:bool)
        n309 = case shown="\"/\"" w472 {
          tunnel: w473 -> [_ w479]
          tunnel: w474 -> [_ w478]
          frame Default {
          }
          frame "/" {
            n310 = call <vilib>:"NT Update Persistence.vi"("Persistence"=w478, "Name"=w479) -> ()  [unwired: 9 in, 1 out]
          }
        }
      }
    }
  }
  n311 = while {
    tunnel: w69 -> [w481]
    i -> [w484]
    stop <- FALSE stop-if-true
    n312 = Wait (ms)(milliseconds to wait=u32 100) -> ()  [unwired: 1 out]
    n313 = case shown="\"Playback\"" "Rec Mode" {
      tunnel: w484 -> [_ _ w499]
      tunnel: [u32 2829099 ("Base Color") u32 11141120 ("Target Color") w488] -> w480
      frame "Stop", Default {
        # "Reset the color, extra updates don't cost much"
      }
      frame "Record" {
      }
      frame "Playback" {
        # "Playback"
        n314 = Quotient & Remainder(x=w499, y=u32 50 ("milliseconds to wait")) -> (x-y*floor(x/y)=w495:u32)  [unwired: 1 out]
        n315 = Divide(x=w495, y=u32 50 ("milliseconds to wait")) -> (x/y=w492:dbl)
        n316 = Multiply(x=6.283185307179586, y=w492) -> (x*y=w497:dbl)
        n317 = Sine(x=w497) -> (sin(x)=w496:dbl)
        n318 = Absolute Value(x=w496) -> (abs(x)=w489:dbl)
        n319 = call "Interpolate RGB Color.vi"("Proportion"=w489, "Target Color"=u32 30976, "Base Color"=u32 2829099) -> ("Result Color"=w488:u32)  [unwired: 8 in]
      }
    }
    n320 = property class="Pane"(reference=w481, "PaneColor"=w480) -> ()  [unwired: 1 in, 2 out]
  }
  n321 = local write "Dashboard Tab"(T2."Drive" ("Dashboard Tab")) -> ()
  n322 = property on="On/Off" class="Bool (strict)"("Visible"=w40) -> ()  [unwired: 2 in, 2 out]
  n323 = property on="Motor" class="Clust (strict)"("Visible"=w40) -> ()  [unwired: 2 in, 2 out]
  n324 = property on="Progress" class="Clust (strict)"("Visible"=w40) -> ()  [unwired: 2 in, 2 out]
  n325 = property on="Test Ring" class="Ring (strict)"("Visible"=w40) -> ()  [unwired: 2 in, 2 out]
  n326 = property on="Rev/Fwd" class="Clust (strict)"("Visible"=w40) -> ()  [unwired: 2 in, 2 out]
  n327 = while {
    tunnel: u16 1741 ("timeout ms (25000)") -> [w501]
    stop <- FALSE stop-if-true
    n328 = TCP Create Listener(10:w501) -> (0:w500:errorcluster, 3:w502:refnum<k5>)  [unwired: 4 in, 1 out]
    n329 = case shown="No Error" w500 {
      selector: w500 -> [w504 _]
      tunnel: w502 -> [w505 _]
      frame No Error {
        n330 = while {
          tunnel: w505 -> [w508]
          tunnel: w504 -> [w507]
          stop <- FALSE stop-if-true
          n331 = TCP Wait On Listener(8:w507, 11:w508) -> (0:w509:errorcluster, 4:w510:refnum<k5>)  [unwired: 2 in, 3 out]
          n332 = local write "TCP"(w510) -> ()
          n333 = case shown="No Error" w509 {
            frame No Error {
            }
            frame Error {
              n334 = Wait (ms)(milliseconds to wait=u32 1000) -> ()  [unwired: 1 out]
            }
          }
        }
      }
      frame Error {
        n335 = Wait (ms)(milliseconds to wait=u32 1000) -> ()  [unwired: 1 out]
      }
    }
  }
  n336 = local write "Command Selection"(u16 0 ("milliseconds to wait")) -> ()
  n337 = local write "Command Params"(string[][] [] ("Command Params")) -> ()
  n338 = global write "WPI_DashboardLogging Global.vi" "Recording"(w63) -> ()
  n339 = local write "Rec Mode"(w63) -> ()
  n340 = call <vilib>:"NT Write String.vi"("String"="Select Auto", "Name"="Auto Selector") -> ()  [unwired: 9 in, 1 out]
  n341 = call-poly <vilib>:"NT Read Value.vi"("Name"="Correct Controller") -> ("String"=→"Controller Verification":string)  [unwired: 9 in, 1 out]
  n342 = call-poly <vilib>:"NT Write Value.vi"("String"="Controller Type", "Name"="Controller Type") -> ()  [unwired: 9 in, 1 out]
